vi "SendAllToZero.vi"(8 "error in (no error)":errorcluster, 11 "VISA resource name":refnum<visa-resource-name>) -> (0 "error out":errorcluster {"code" format="%.0x"}, 3 "VISA resource name out":refnum<visa-resource-name>)   [LabVIEW 2015]
uses:
  <userlib>/Newport ESP301/Newport ESP301.lvlib
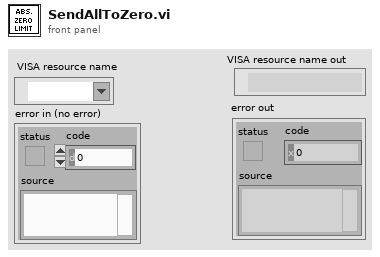
[diagram p1: front panel]
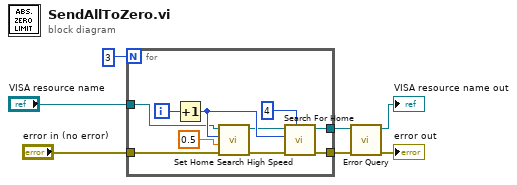
[diagram p0: block diagram]
diagram:
  n1 = for {
    N: 3 -> [_]
    tunnel: "VISA resource name" -> [w15]
    tunnel: [w12] -> w3
    tunnel: [w11] -> w2
    tunnel: "error in (no error)" -> [w9]
    i -> [w17]
    n2 = Increment(x=w17) -> (x+1=w16:i32)
    n3 = call <userlib>:"Set Home Search High Speed.vi"("error in (no error)"=w9, "Search High Speed (0 units/s)"=0.5, "Axis (1)"=w16, "VISA resource name"=w15) -> ("error out"=w13:errorcluster, "VISA resource name out"=w14:refnum<visa-resource-name>)  [unwired: 2 in]
    n4 = call <userlib>:"Search For Home.vi"("Home mode"=4, "error in (no error)"=w13, "Axis (1)"=w16, "VISA resource name"=w14) -> ("error out"=w12:errorcluster, "VISA resource name out"=w11:refnum<visa-resource-name>)  [unwired: 3 in]
  }
  n5 = call <userlib>:"Error Query.vi"("error in (no error)"=w3, "VISA resource name"=w2) -> ("error out"=→"error out":errorcluster, "VISA resource name out"=→"VISA resource name out":refnum<visa-resource-name>)  [unwired: 2 in, 2 out]
